vi "_VI Missing or Broken.vi"(11 "Path":path) -> (3 "missing or broken?":bool)   [LabVIEW 2017, in "interfacebrowser.lvlib"]
uses:
  interfacebrowser.lvlib
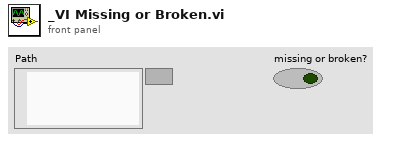
[diagram p1: front panel]
types:
  T1 = enum32{"Bad", "Idle", "Run top level", "Running"}
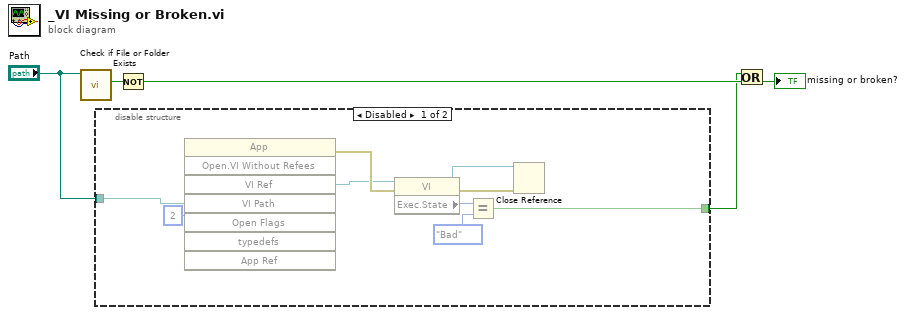
[diagram p0: block diagram]
diagram:
  n1 = call <vilib>:"Check if File or Folder Exists.vi"("path"="Path") -> ("file or folder exists?"=w5:bool)  [unwired: 8 in, 2 out]
  n2 = disable-structure shown="Disabled" {
    disable-tunnel: "Path" -> [w14 _]
    disable-tunnel: [w7 _] -> w1
    frame Disabled {
      n3 = invoke class="App" method="Open.VI Without Refees"("VI Path"=w14, "Open Flags"=2) -> (error out=w11:errorcluster, "VI Ref"=w6:refnum<vi>)  [unwired: 6 in, 6 out]
      n4 = property class="VI"(reference=w6, error in=w11) -> (reference out=w12:refnum<vi>, error out=w10:errorcluster, "Exec.State"=w9:T1)
      n5 = Equal?(x=w9, y=T1."Bad") -> (x = y?=w7:bool)
      n6 = Close Reference(reference=w12, error in (no error)=w10) -> ()  [unwired: 1 out]
    }
    frame Enabled {
      # "if check borken, it will be slow"
    }
  }
  n7 = Not(x=w5) -> (.not. x?=w4:bool)
  n8 = Or(x=w1, y=w4) -> (x .or. y?=→"missing or broken?":bool)
